vi "Select Str.vi"(0 "DB Path":string, 1 "Where Clause":string, 5 "Include RowID":bool, 9 "Tables Name":string, 11 "error in (no error)":errorcluster, 12 "Columns":string[](array[string]), 13 "Distinct":bool) -> (3 "Results":string[][](array[string]), 4 "DB Path Out":string, 10 "Table Name Out":string, 15 "error out":errorcluster)   [LabVIEW 2016]
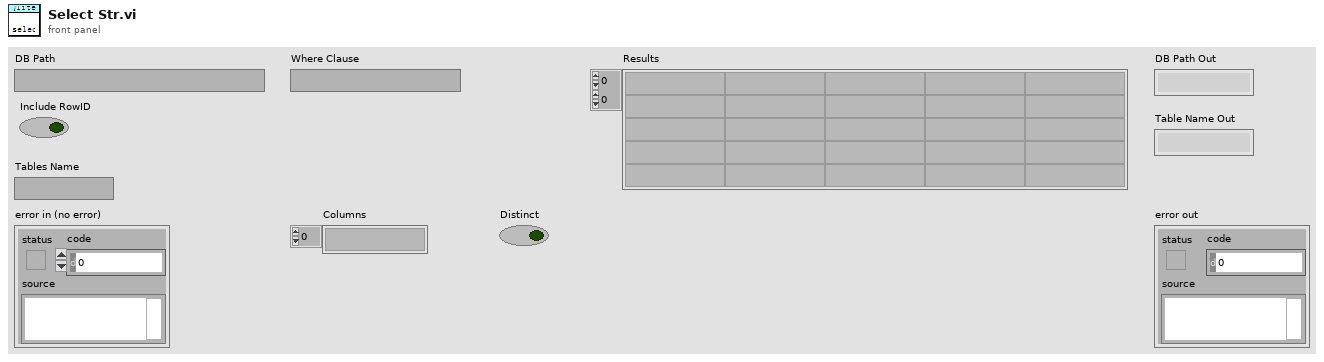
[diagram p1: front panel]
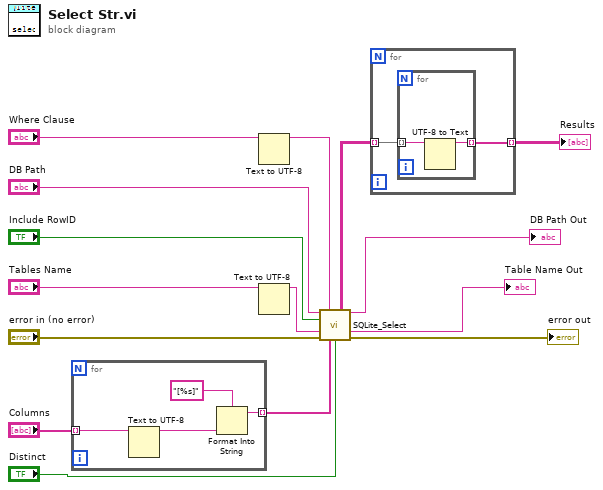
[diagram p0: block diagram]
diagram:
  n1 = for {
    tunnel: "Columns" -> [w19] mode=indexing
    tunnel: [w17] -> w13 mode=indexing
    n2 = Text to UTF-8(11:w19) -> (3:w18:string)  [unwired: 2 in, 1 out]
    n3 = Format Into String(format string="[%s]" ("格式字符串"), w18) -> (resulting string=w17:string)  [unwired: 2 in, 1 out]
  }
  n4 = Text to UTF-8(11:"Where Clause") -> (3:w11:string)  [unwired: 2 in, 1 out]
  n5 = Text to UTF-8(11:"Tables Name") -> (3:w9:string)  [unwired: 2 in, 1 out]
  n6 = call-poly <userlib>:"SQLite_Select.vi"("DB Path"="DB Path", "Where Clause"=w11, "Include RowID"="Include RowID", "Table Name"=w9, "error in (no error)"="error in (no error)", "Columns"=w13, "Distinct"="Distinct") -> ("Results"=w14:string[][], "DB Path Out"=→"DB Path Out":string, "Table Name Out"=→"Table Name Out":string, "error out"=→"error out":errorcluster)  [unwired: 5 in]
  n7 = for {
    tunnel: w14 -> [w21] mode=indexing
    tunnel: [w20] -> w15 mode=indexing
    n8 = for {
      tunnel: w21 -> [w22] mode=indexing
      tunnel: [w23] -> w20 mode=indexing
      n9 = UTF-8 to Text(11:w22) -> (3:w23:string)  [unwired: 2 in, 1 out]
    }
  }
  "Results" <- w15
